vi "Simulation check.vi"(11 "error in (no error)":errorcluster) -> (3 "Error":bool)   [LabVIEW 2020]
uses:
  <vilib>/Utility/error.llb/DialogType.ctl
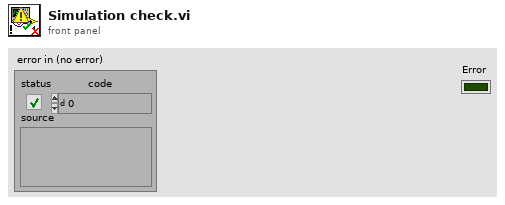
[diagram p1: front panel]
types:
  T1 = typedef "DialogType.ctl" = u16
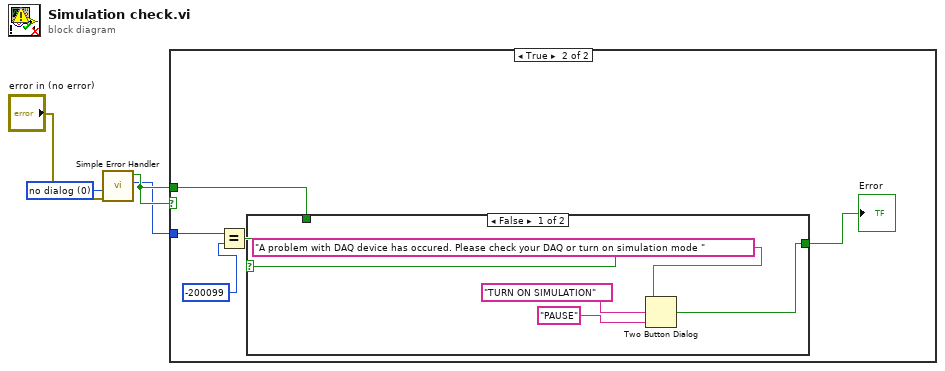
[diagram p0: block diagram]
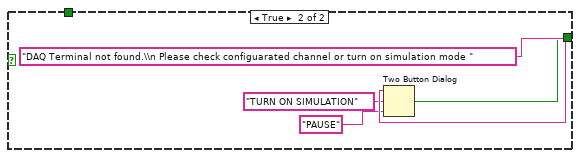
[diagram p3: hidden frame]
diagram:
  w1 = T1 0 items=["no dialog", "OK message", "continue or stop message", "OK message + warnings", "continue/stop + warnings"] ("type of dialog (OK msg:1)")
  n1 = call <vilib>:"Simple Error Handler.vi"("type of dialog (OK msg:1)"=w1, "error in (no error)"="error in (no error)") -> ("error?"=w3:bool, "code out"=w2:i32)  [unwired: 3 in, 3 out]
  n2 = case shown="True" w3 {
    tunnel: w3 -> [_ w5]
    tunnel: w2 -> [_ w9]
    frame False {
    }
    frame True {
      n3 = Equal?(x=w9, y=-200099) -> (x = y?=w7:bool)
      n4 = case shown="False" w7 {
        tunnel: [w10 w14] -> w6
        tunnel: w5 -> [_ _]
        frame False {
          n5 = Two Button Dialog(message="A problem with DAQ device has occured. Please check your DAQ or turn on simulation mode ", 1:"PAUSE" ("button name (\"OK\")"), 2:"TURN ON SIMULATION" ("T button name (\"OK\")")) -> (T button?=w10:bool)
        }
        frame True {
          n6 = Two Button Dialog(message="DAQ Terminal not found.\\n Please check configuarated channel or turn on simulation mode ", 1:"PAUSE" ("button name (\"OK\")"), 2:"TURN ON SIMULATION" ("T button name (\"OK\")")) -> (T button?=w14:bool)
        }
      }
      "Error" <- w6
    }
  }
